vi "Get Collatz sequence-with array output.vi"(8 "error in (no error)":errorcluster, 11 "n":u64) -> (0 "error out":errorcluster, 1 "T = U64 overflow\nsequence has not ended":bool, 2 "no. of elements (chain length)":i32, 3 "Collatz sequence of n":u64[](array[numeric]))   [LabVIEW 2021, in "Numeric Utilities.lvlib"]
doc: "Warning: This VI runs out of memory for some values of n."
uses:
  Numeric Utilities.lvlib
panel:
  out "max value":u64
  out "Collatz sequence":u64[](graph)
  in  "Dev: stop early":bool
  out "iteration":i32
  # "Development\ncontrols/indicators useful for development and testing, but which are not outputs of the VI"
  # "Input\nInputs to the VI"
  # "Output\nOutputs of the VI"
  # "Description\n\nWarning: This VI runs out of memory for some values of n."
  # "113383"
  # "when n = 837,799"
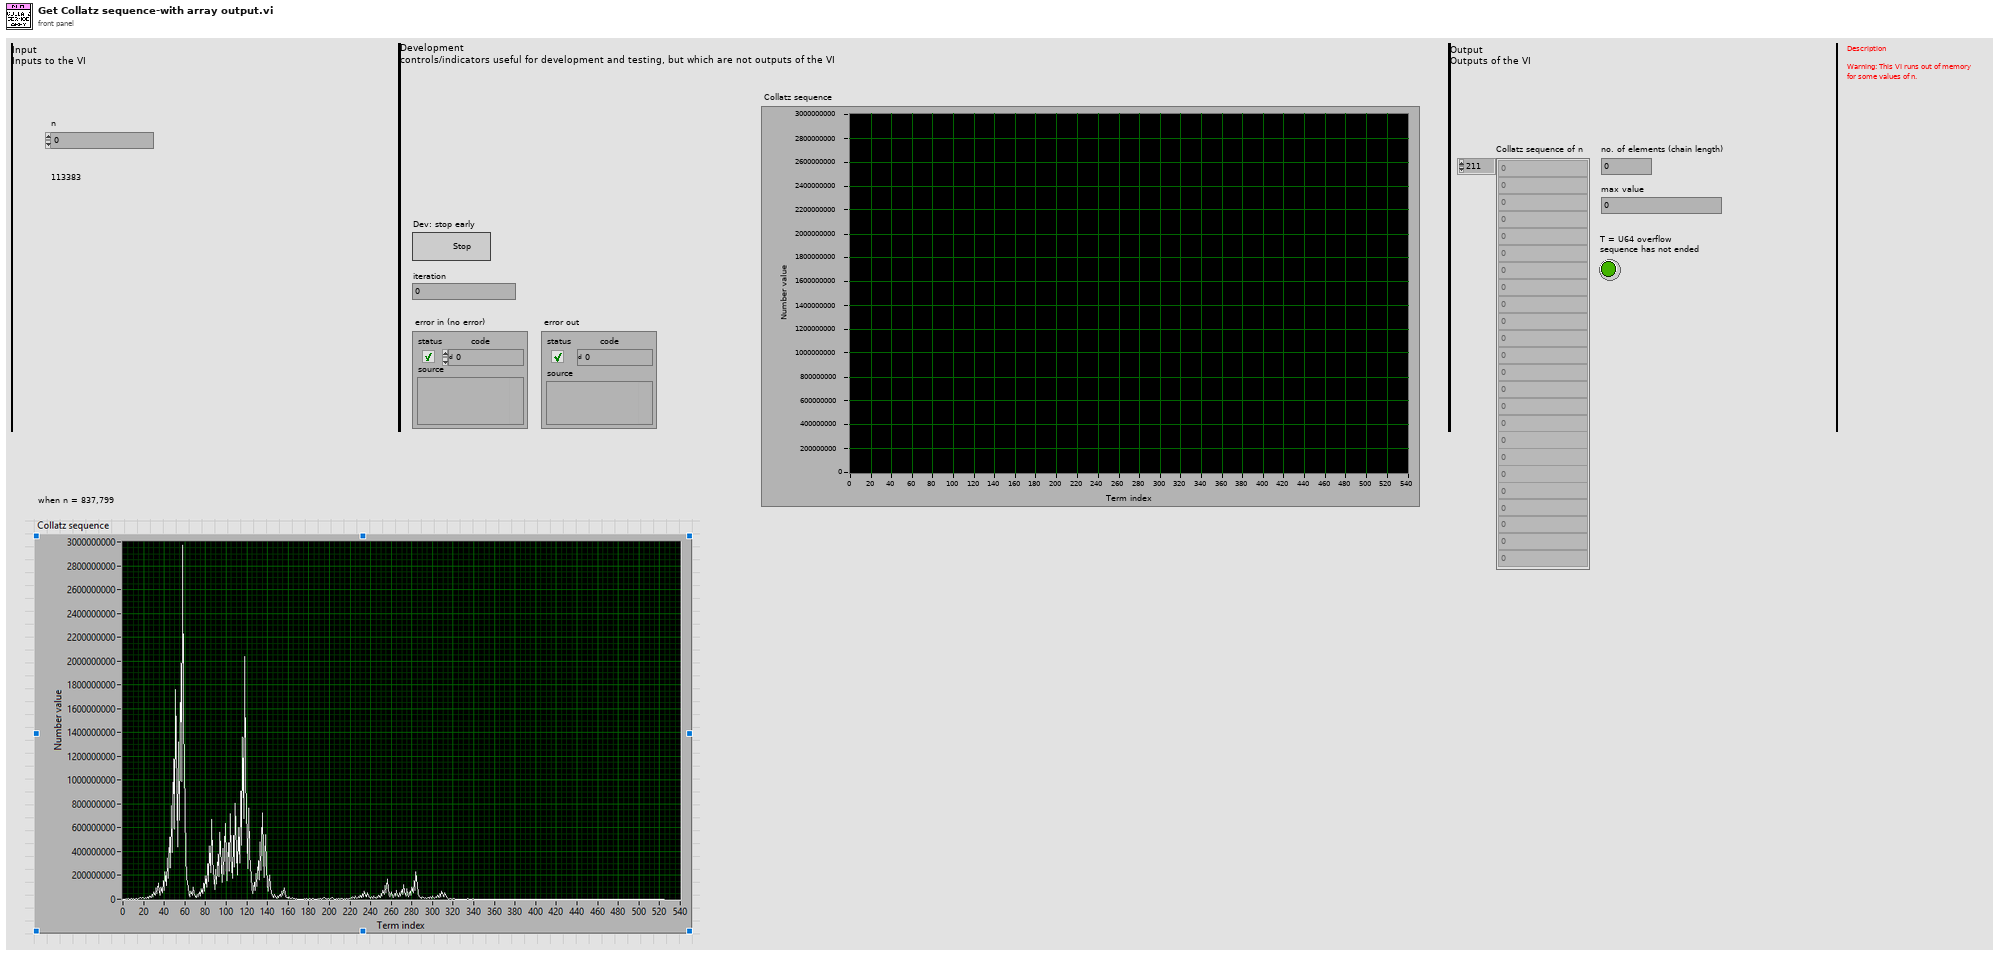
[diagram p1: front panel]
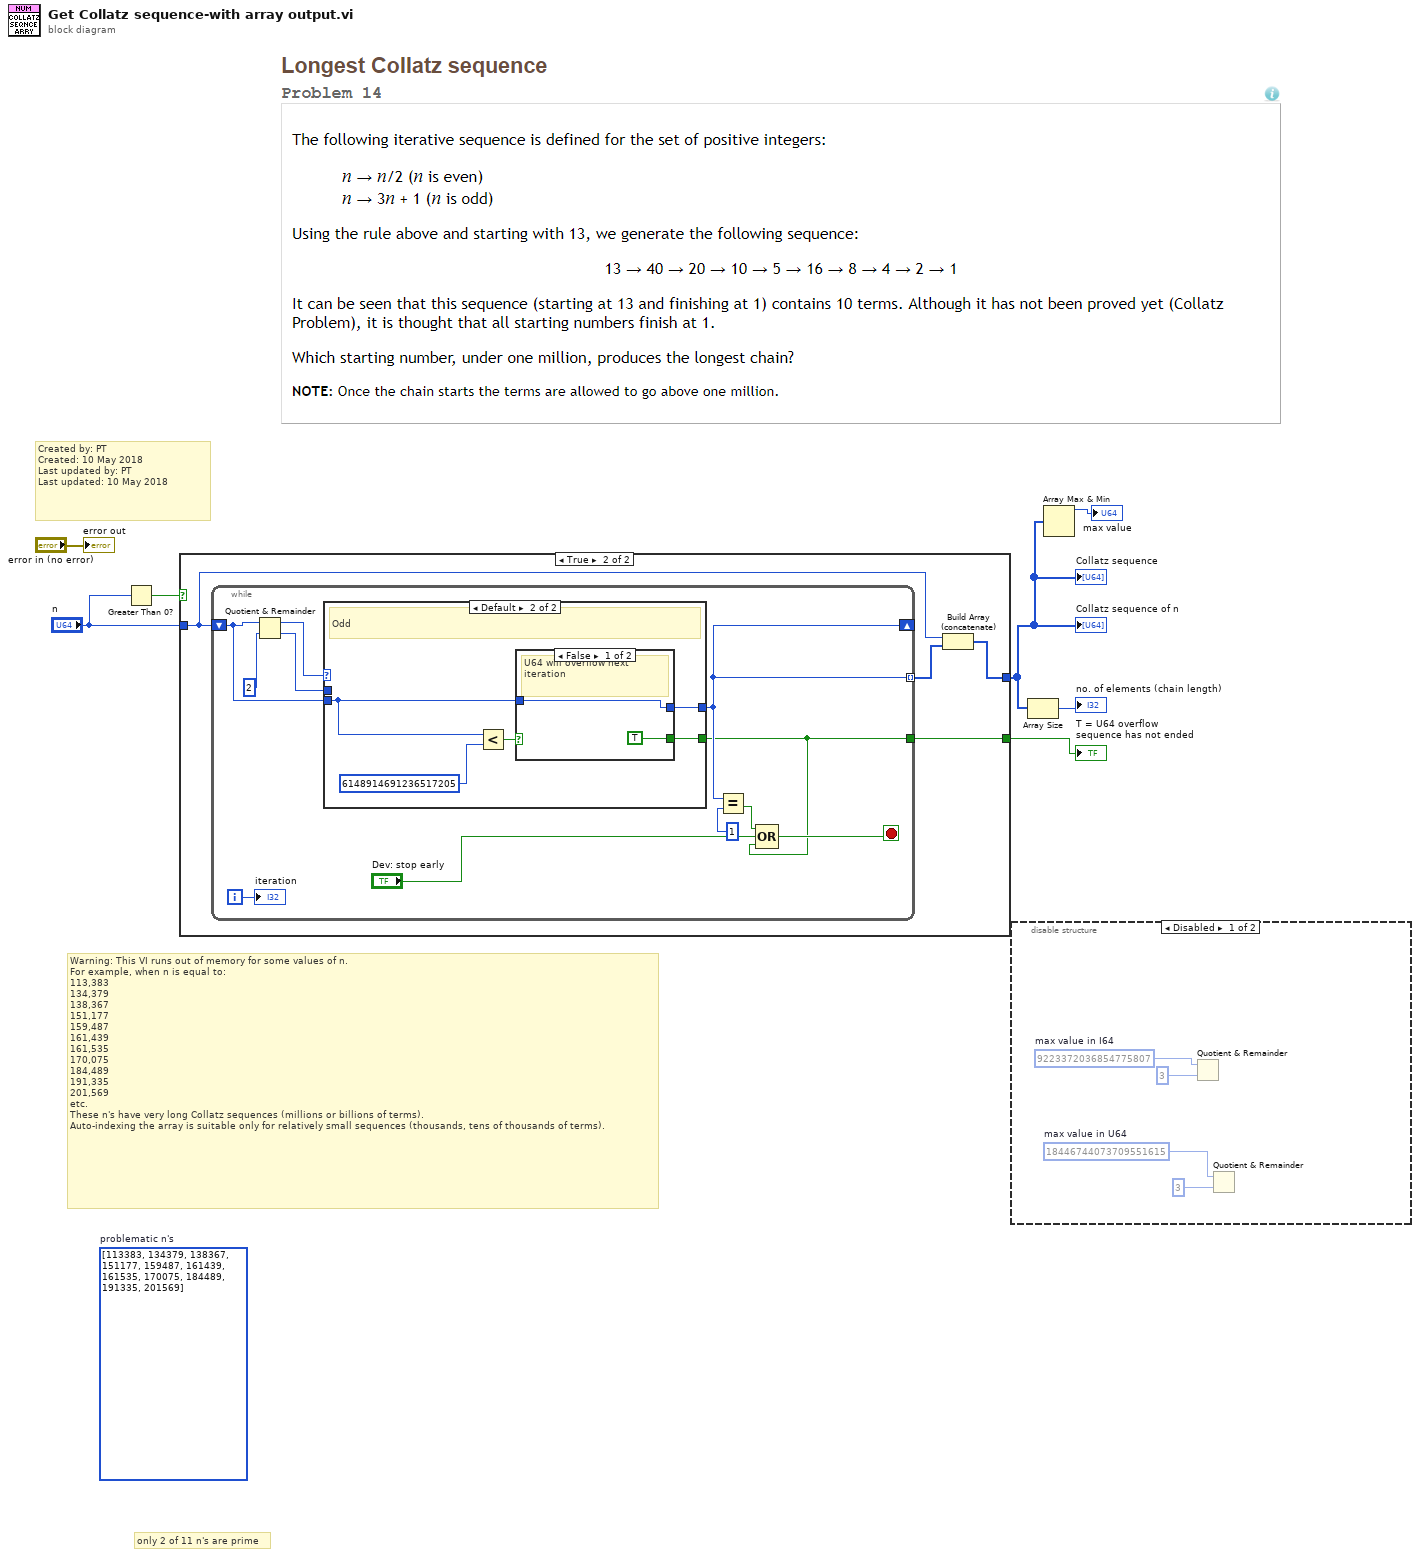
[diagram p0: block diagram]
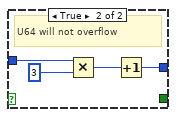
[diagram p5: hidden frame]
diagram:
  (unwired) i64[] [113383, 134379, 138367, 151177, 159487, 161439, 161535, 170075, 184489, 191335, 201569]  # problematic n's
  # "only 2 of 11 n's are prime"
  # "Warning: This VI runs out of memory for some values of n. \nFor example, when n is equal to:\n113,383\n134,379\n138,367\n151,177\n159,487\n161,439\n161,535\n170,075\n184,489\n191,335\n201,569\netc.\nThese n's have very long Collatz sequences (millions or billions of terms). \nAuto-indexing the array is suitable only for relatively small sequences (thousands, tens of thousands of terms)."
  # "Created by: PT\nCreated: 10 May 2018\nLast updated by: PT\nLast updated: 10 May 2018"
  n1 = Greater Than 0?(x="n") -> (x > 0?=w6:bool)
  n2 = case shown="True" w6 {
    tunnel: "n" -> [_ w9]
    tunnel: [_ w10] -> w3
    tunnel: [_ w8] -> w1
    frame False {
    }
    frame True {
      n3 = while {
        shift-right: [w18] -> _
        shift-left: w9 -> [w16]
        tunnel: [w18] -> w11 mode=indexing
        tunnel: [w12] -> w8
        i -> [w21]
        stop <- w17 stop-if-true
        n4 = Quotient & Remainder(x=w16, y=u64 2) -> (x-y*floor(x/y)=w14:u64, floor(x/y)=w13:u64)
        n5 = case shown="Default" w14 {
          tunnel: w16 -> [_ w27]
          tunnel: [w23 w28] -> w18
          tunnel: w13 -> [w23 _]
          tunnel: [_ w24] -> w12
          frame 0 {
            # "Even"
          }
          frame Default {
            # "Odd"
            n6 = Less?(x=w27, y=u64 6148914691236517205) -> (x < y?=w25:bool)
            n7 = case shown="False" w25 {
              tunnel: [w30 w32] -> w28
              tunnel: w27 -> [w30 w31]
              tunnel: [TRUE _] -> w24
              frame False {
                # "U64 will overflow next iteration"
              }
              frame True {
                # "U64 will not overflow"
                n8 = Multiply(x=w31, y=u64 3) -> (x*y=w33:u64)
                n9 = Increment(x=w33) -> (x+1=w32:u64)
              }
            }
          }
        }
        n10 = Equal?(x=w18, y=u64 1) -> (x = y?=w20:bool)
        n11 = Compound Arithmetic op=OR(w20, "Dev: stop early", w12) -> (w17:bool)
        "iteration" <- w21
      }
      n12 = Build Array (concatenate)(w9, w11) -> (w10:u64[])
    }
  }
  "Collatz sequence of n" <- w3
  "Collatz sequence" <- w3
  "T = U64 overflow\nsequence has not ended" <- w1
  n13 = disable-structure shown="Disabled" {
    frame Disabled {
      w36 = u64 18446744073709551615  # max value in U64
      w40 = i64 9223372036854775807  # max value in I64
      n14 = Quotient & Remainder(x=w40, y=i64 3) -> (floor(x/y)=w38:i64)  [unwired: 1 out]
      n15 = Quotient & Remainder(x=w36, y=u64 3) -> (floor(x/y)=w35:u64)  [unwired: 1 out]
    }
    frame Enabled {
    }
  }
  n16 = Array Size(array=w3) -> (size(s)=→"no. of elements (chain length)":i32)
  n17 = Array Max & Min(array=w3) -> (max value=→"max value":u64)  [unwired: 3 out]
  "error out" <- "error in (no error)"
